vi "Read Shield Count.vi"(8 "error in (no error)":errorcluster, 11 "Shield in":refnum<class "Shield.lvclass">) -> (0 "error out":errorcluster, 2 "Shield Count":u8, 3 "Shield out":refnum<class "Shield.lvclass">)   [LabVIEW 2021, in "Shield.lvclass"]
uses:
  Shield.lvclass
  Shield.lvclass/Shield.ctl
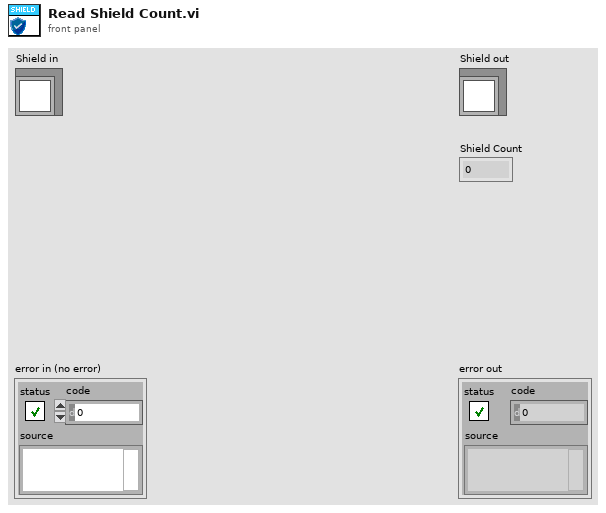
[diagram p1: front panel]
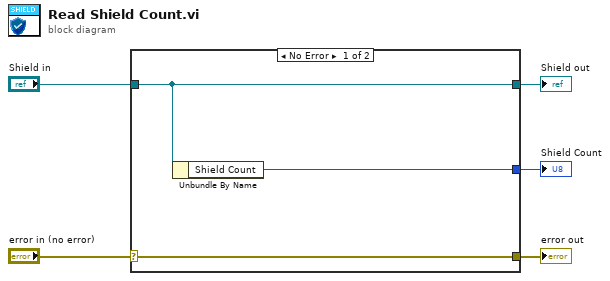
[diagram p0: block diagram]
diagram:
  n1 = case shown="No Error" "error in (no error)" {
    selector: "error in (no error)" -> [w8 w9]
    tunnel: [w8 w9] -> w4
    tunnel: [w7 w10] -> w2
    tunnel: "Shield in" -> [w7 w10]
    tunnel: [w6 _] -> w1
    frame No Error {
      n2 = Unbundle By Name(w7) -> ("Shield Count"=w6:u8)
    }
    frame Error {
    }
  }
  "error out" <- w4
  "Shield out" <- w2
  "Shield Count" <- w1
